vi "Resideo Get All Vesta Data.vi"(8 "error in (no error)":errorcluster, 11 "Modbus Master in":refnum<class "Modbus Master.lvclass">) -> (0 "error out":errorcluster, 2 "Vesta Data Output":T1, 3 "Modbus Master out":refnum<class "Modbus Master.lvclass">)   [LabVIEW 2020]
uses:
  Type Definitions/Vesta Info.ctl
  <vilib>/NI/Modbus Library/API/Master/Modbus Master.lvclass
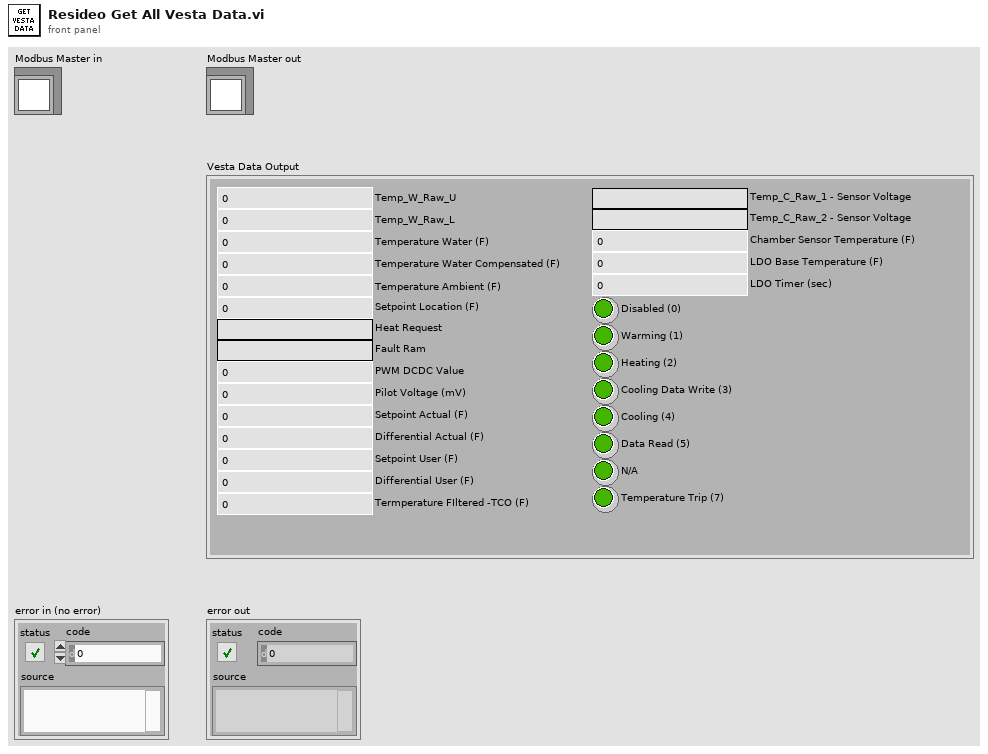
[diagram p1: front panel]
types:
  T1 = typedef "Vesta Info.ctl" = cluster{"Temp_W_Raw_U":u16, "Temp_W_Raw_L":u16, "Temperature Water (F)":dbl, "Temperature Water Compensated (F)":dbl, "Temperature Ambient (F)":dbl, "Setpoint Location (F)":dbl, "Heat Request":string, "Fault Ram":string, "PWM DCDC Value":u16, "Pilot Voltage (mV)":dbl, "Setpoint Actual (F)":dbl, "Differential Actual (F)":dbl, "Setpoint User (F)":dbl, "Differential User (F)":dbl, "Termperature FIltered -TCO (F)":dbl, "Temp_C_Raw_1 - Sensor Voltage":string, "Temp_C_Raw_2 - Sensor Voltage":string, "Chamber Sensor Temperature (F)":dbl, "LDO Base Temperature (F)":dbl, "LDO Timer (sec)":i16, "Disabled (0)":bool, "Warming (1)":bool, "Heating (2)":bool, "Cooling Data Write (3)":bool, "Cooling (4)":bool, "Data Read (5)":bool, "N/A":bool, "Temperature Trip (7)":bool}
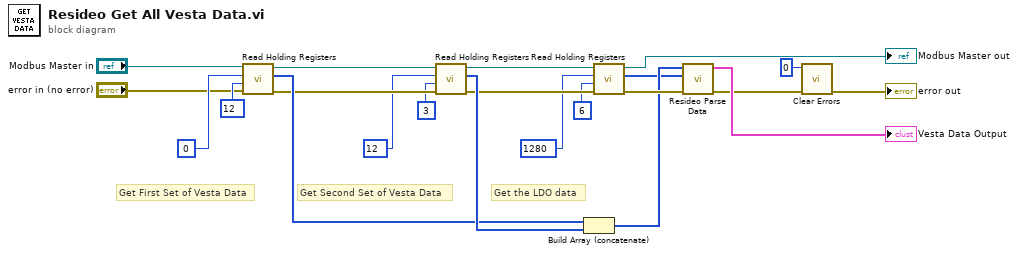
[diagram p0: block diagram]
diagram:
  # "Get Second Set of Vesta Data"
  # "Get First Set of Vesta Data"
  # "Get the LDO data"
  n1 = call-dynamic "Read Holding Registers.vi"("error in"="error in (no error)", "number of inputs"=12 ("Register"), "starting address"=u16 0, "Modbus master in"="Modbus Master in") -> ("error out"=w15:errorcluster, "register values"=w18:u16[], "Modbus master out"=w14:refnum<class "Modbus Master.lvclass">)  [unwired: 5 in]
  n2 = call-dynamic "Read Holding Registers.vi"("error in"=w15, "number of inputs"=3 ("Register"), "starting address"=u16 12, "Modbus master in"=w14) -> ("error out"=w17:errorcluster, "register values"=w19:u16[], "Modbus master out"=w16:refnum<class "Modbus Master.lvclass">)  [unwired: 5 in]
  n3 = Build Array (concatenate)(w18, w19) -> (w20:u16[])
  n4 = call-dynamic "Read Holding Registers.vi"("error in"=w17, "number of inputs"=6 ("Register"), "starting address"=u16 1280, "Modbus master in"=w16) -> ("error out"=w21:errorcluster, "register values"=w10:u16[], "Modbus master out"=→"Modbus Master out":refnum<class "Modbus Master.lvclass">)  [unwired: 5 in]
  n5 = call "Resideo Parse Data.vi"("error in (no error)"=w21, "LDO Data"=w10, "Vesta Data 1"=w20) -> ("error out"=w3:errorcluster, "Vesta Data Output"=→"Vesta Data Output":T1)  [unwired: 7 in]
  n6 = call <vilib>:"Clear Errors.vi"("error in (no error)"=w3, "specific error code to clear (0: all)"=0) -> ("error out"=→"error out":errorcluster)  [unwired: 4 in, 1 out]
